vi "example of p13-1.vi"() -> ()   [LabVIEW 2017]
panel:
  out "XY Graph 2":cluster{"Y":dbl[], "Y":dbl[]}[](graph)
  out "decimated array 2":i32[](array[numeric])
  out "decimated array":i32[](array[numeric])
  out "XY Graph":cluster{"Y":dbl[], "Y":dbl[]}[](graph)
  out "y":i32[](array[numeric])
  out "x":i32[](array[numeric])
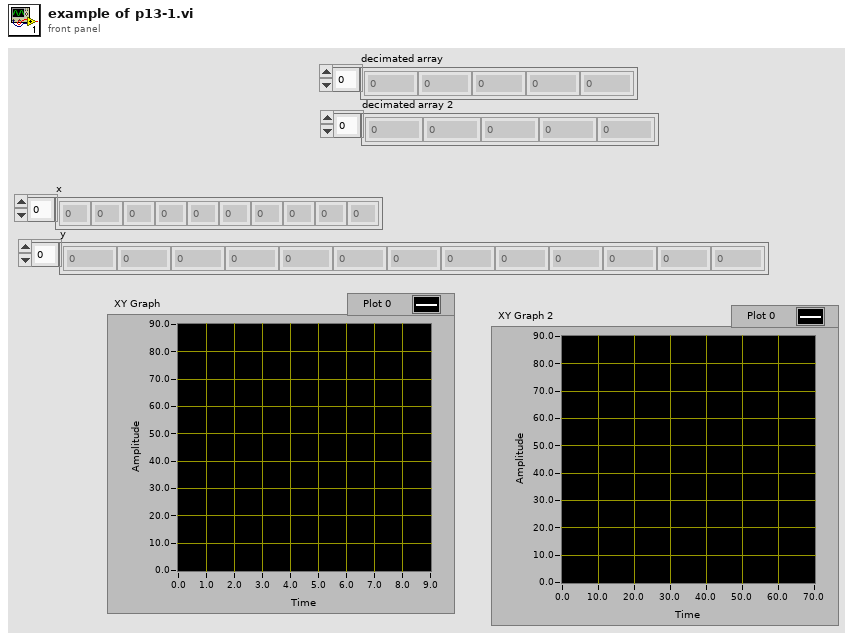
[diagram p1: front panel]
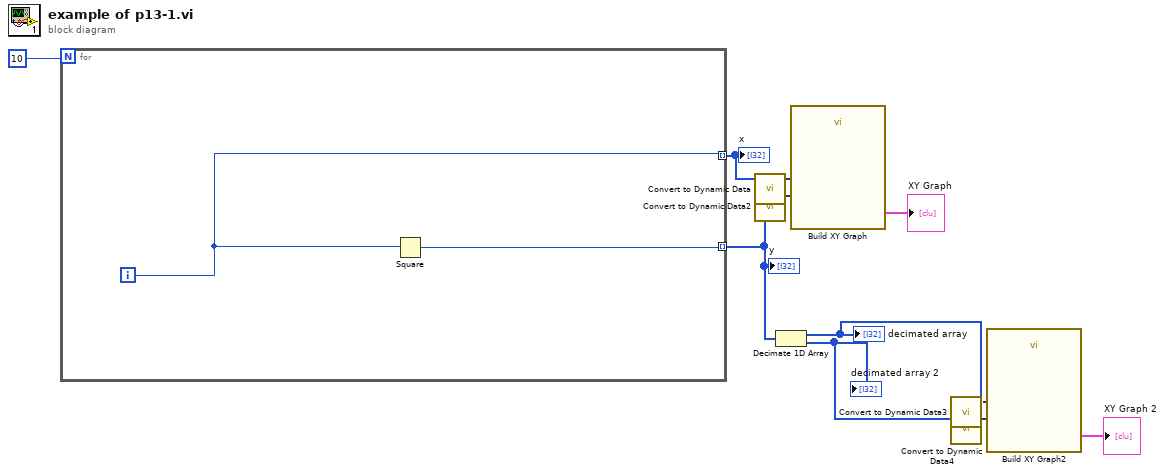
[diagram p0: block diagram]
diagram:
  n1 = for {
    N: 10 -> [_]
    tunnel: [w13] -> w9 mode=indexing
    tunnel: [w12] -> w6 mode=indexing
    i -> [w13]
    n2 = Square(x=w13) -> (x^2=w12:i32)
  }
  "x" <- w9
  "y" <- w6
  n3 = call "Convert to Dynamic Data"("Array"=w9) -> ("Dynamic Data Type"=w8:dynamicdata)  [unwired: 3 in]
  n4 = call "Convert to Dynamic Data2"("Array"=w6) -> ("Dynamic Data Type"=w7:dynamicdata)  [unwired: 3 in]
  n5 = Decimate 1D Array(w6) -> (w4:i32[], w2:i32[])
  "decimated array" <- w4
  "decimated array 2" <- w2
  n6 = call "Build XY Graph"("Y Input"=w7, "X Input"=w8) -> ("XY Graph"=→"XY Graph":cluster{"X":dbl[], "Y":dbl[]}[])  [unwired: 8 in, 1 out]
  n7 = call "Convert to Dynamic Data3"("Array"=w4) -> ("Dynamic Data Type"=w3:dynamicdata)  [unwired: 3 in]
  n8 = call "Convert to Dynamic Data4"("Array"=w2) -> ("Dynamic Data Type"=w1:dynamicdata)  [unwired: 3 in]
  n9 = call "Build XY Graph2"("Y Input"=w1, "X Input"=w3) -> ("XY Graph"=→"XY Graph 2":cluster{"X":dbl[], "Y":dbl[]}[])  [unwired: 8 in, 1 out]
